vi "SortThresholdCfg.vi"(7 "RX?":bool=TRUE, 11 "TC13":T2 {"ErrsAndWarns" scale=0.0..10.0}) -> (3 "ThresholdCluster":T1={"Enable"=FALSE, "LoErr"=0.0, "LoWarn"=0.0, "HiWarn"=0.0, "HiErr"=0.0, "RX?"=TRUE})   [LabVIEW 2018]
uses:
  Controls/Clusts/AlarmThresh_OneChan.ctl
  Controls/Clusts/ThresholdAlarmLimits.ctl
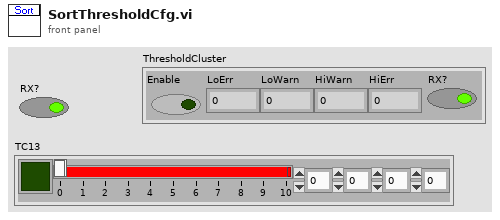
[diagram p1: front panel]
types:
  T1 = typedef "ThresholdAlarmLimits.ctl" = cluster{"Enable":bool, "LoErr":dbl, "LoWarn":dbl, "HiWarn":dbl, "HiErr":dbl, "RX?":bool}
  T2 = typedef "AlarmThresh_OneChan.ctl" = cluster{"Enbl":bool, "ErrsAndWarns":cluster{dbl, dbl, dbl, dbl}}
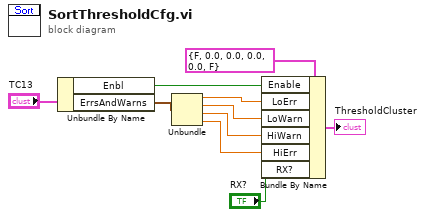
[diagram p0: block diagram]
diagram:
  n1 = Unbundle By Name("TC13") -> ("Enbl"=w4:bool, "ErrsAndWarns"=w5:cluster{dbl, dbl, dbl, dbl})
  n2 = Unbundle(w5) -> (w6:dbl, w7:dbl, w8:dbl, w9:dbl)
  n3 = Bundle By Name(cluster=T1 {"Enable"=FALSE, "LoErr"=0.0, "LoWarn"=0.0, "HiWarn"=0.0, "HiErr"=0.0, "RX?"=FALSE} ("Thresholds"), "Enable"=w4, "LoErr"=w6, "LoWarn"=w7, "HiWarn"=w8, "HiErr"=w9, "RX?"="RX?") -> (→"ThresholdCluster":T1)
